vi "QDM matlab saver.vi"(4 "numFreqs":i32=51, 6 "img data stack Input":dbl[][](array[numeric]), 7 "matlab path":path, 8 "Height":i64(slide)=1200 min=0 max=1200 step=4 scale=0.0..1200.0, 9 "Width":i64(slide)=1920 min=0 max=1920 step=4 scale=0.0..1920.0, 10 "freq list (Hz)":dbl[](array[numeric]), 11 "sweep #":i32) -> ()   [LabVIEW 2018]
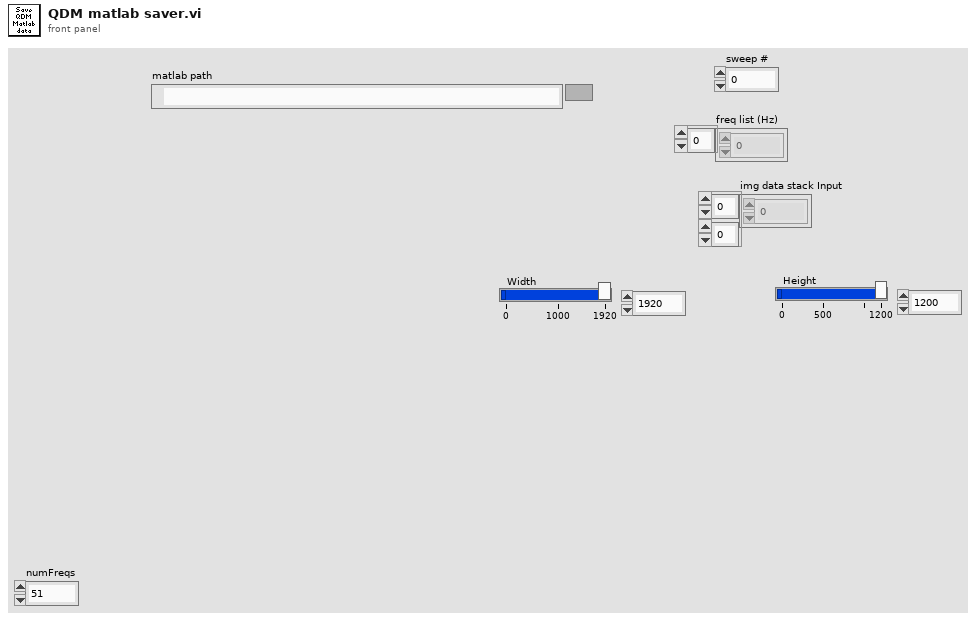
[diagram p1: front panel]
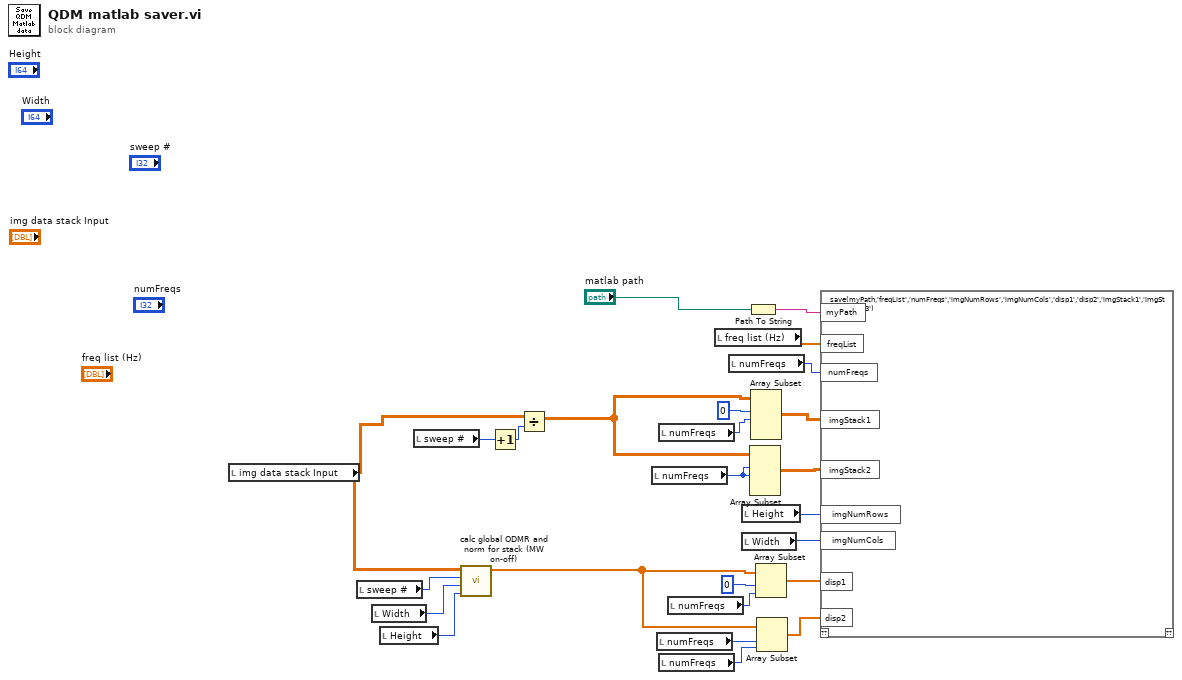
[diagram p0: block diagram]
diagram:
  n1 = local read "img data stack Input"() -> (w3:dbl[][])
  n2 = local read "sweep #"() -> (w4:i32)
  n3 = local read "Width"() -> (w8:i64)
  n4 = local read "Height"() -> (w9:i64)
  n5 = local read "sweep #"() -> (w6:i32)
  n6 = call "calc global ODMR and norm for stack (MW on-off).vi"("Height"=w9, "Width"=w8, "sweep #"=w4, "img data stack"=w3) -> ("normed spectrum"=w7:dbl[])  [unwired: 7 in]
  n7 = Increment(x=w6) -> (x+1=w5:i32)
  n8 = Divide(x=w3, y=w5) -> (x/y=w2:dbl[][])
  n9 = local read "numFreqs"() -> (w11:i32)
  n10 = local read "numFreqs"() -> (w18:i32)
  n11 = local read "numFreqs"() -> (w13:i32)
  n12 = local read "numFreqs"() -> (w17:i32)
  n13 = local read "numFreqs"() -> (w19:i32)
  n14 = local read "freq list (Hz)"() -> (w24:dbl[])
  n15 = local read "numFreqs"() -> (w23:i32)
  n16 = local read "Height"() -> (w21:i64)
  n17 = local read "Width"() -> (w22:i64)
  n18 = Path To String(path="matlab path") -> (string=w25:string)
  n19 = Array Subset(array=w2, index (row)=w11, length (row)=w11) -> (w10:dbl[][])  [unwired: 2 in]
  n20 = Array Subset(array=w2, index (row)=0 ("index"), length (row)=w13) -> (w12:dbl[][])  [unwired: 2 in]
  n21 = Array Subset(array=w7, index=0, length=w19) -> (w16:dbl[])
  n22 = Array Subset(array=w7, index=w18, length=w17) -> (w15:dbl[])
  n23 = script code="save(myPath,'freqList','numFreqs','imgNumRows','imgNumCols','disp1','disp2','imgStack1','imgStack2','-v7.3')"("myPath"=w25, "freqList"=w24, "imgStack1"=w12, "numFreqs"=w23, "imgNumRows"=w21, "imgNumCols"=w22, "disp1"=w16, "disp2"=w15, "imgStack2"=w10) -> ()  [unwired: 1 in, 1 out]
